vi "Action-engine-wrapper-example.vi"(7 "Action":T2(ring), 8 "error in (no error)":errorcluster, 9 "Additional message":string, 10 "Custom error":T1=enum."State not implemented") -> (0 "error out":errorcluster)   [LabVIEW 2013, in "Error-handling.lvlib" / "Errors.lvclass"]
uses:
  Errors.lvclass
  Custom-errors.ctl
  Settings.ctl
  Languages.ctl
  Ignore-error-custom.vi
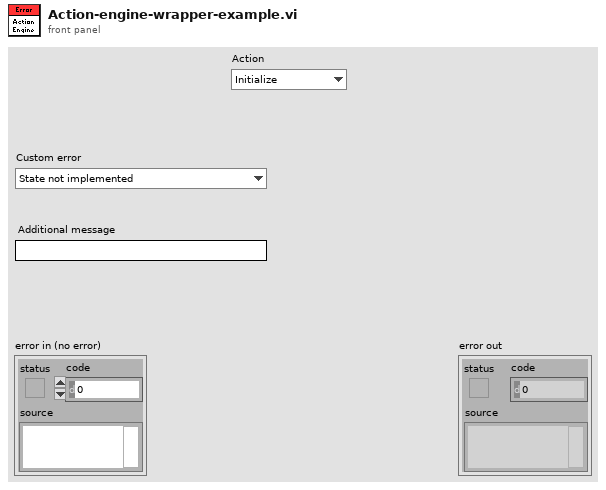
[diagram p1: front panel]
types:
  T1 = typedef "Error-handling.lvlib/Errors.lvclass/Custom-errors.ctl" = enum16{"No error", "State not implemented", "Initialization failed", "Language not implemented", "Error not implemented"}
  T2 = enum16{"Initialize", "Ignore", "Invoke", "Process", "Clear"}
  T3 = typedef "Error-handling.lvlib/Errors.lvclass/Settings.ctl" = cluster{"Language":T4, "Display error dialog":bool, "Write log to file":bool, "Stream to log file":bool, "Overwrite existing log":bool, "Max log size":i32, "Max number of log files":i32}
  T4 = typedef "Error-handling.lvlib/Errors.lvclass/Languages.ctl" = enum16{"English"}
  T5 = typedef "Error-handling.lvlib/Errors.lvclass/Object-reference.ctl" = refnum<data-value>
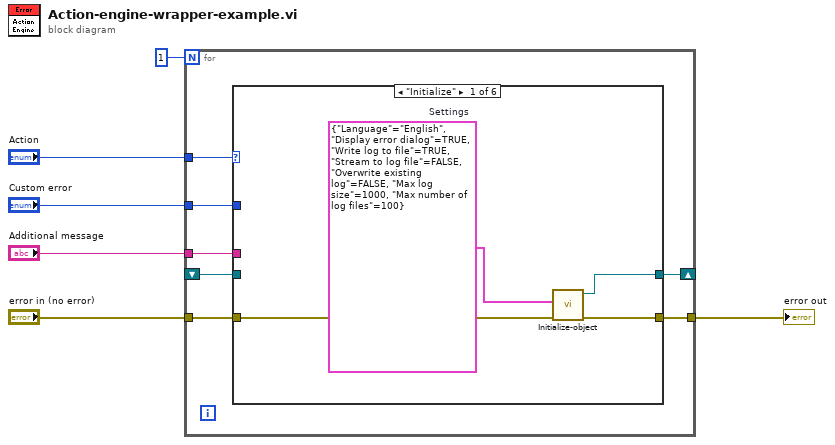
[diagram p0: block diagram]
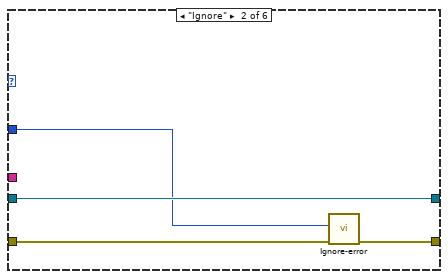
[diagram p2: hidden frame]
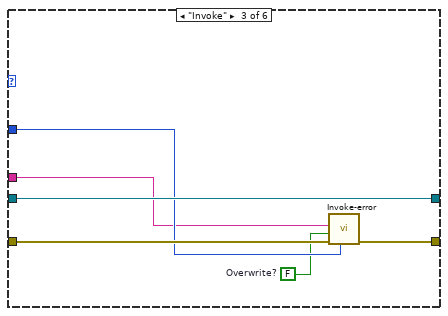
[diagram p3: hidden frame]
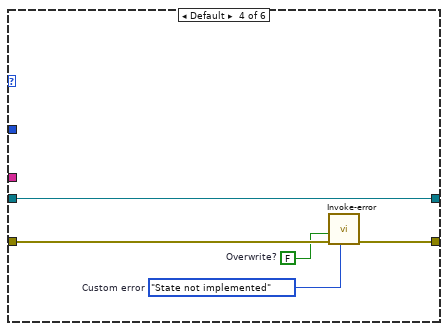
[diagram p4: hidden frame]
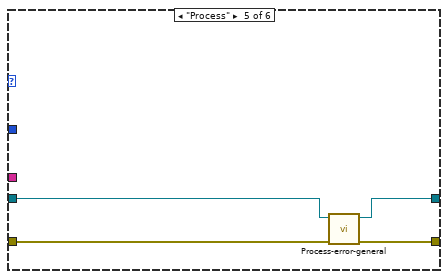
[diagram p5: hidden frame]
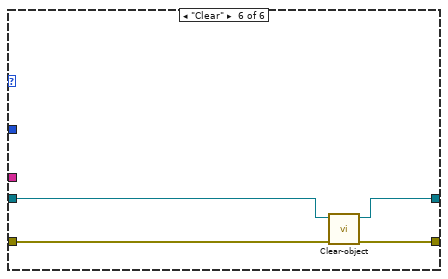
[diagram p6: hidden frame]
diagram:
  n1 = for {
    N: 1 -> [_]
    tunnel: "error in (no error)" -> [w10]
    tunnel: "Action" -> [w13]
    tunnel: "Custom error" -> [w12]
    tunnel: "Additional message" -> [w11]
    tunnel: [w9] -> w1
    shift-right: [w8] -> _
    shift-left: _ -> [w7]
    n2 = case shown="\"Initialize\"" w13 {
      tunnel: w12 -> [_ w18 w24 _ _ _]
      tunnel: w11 -> [_ _ w23 _ _ _]
      tunnel: w10 -> [w17 w19 w25 w30 w35 w39]
      tunnel: [w16 w21 w27 w32 w36 w40] -> w9
      tunnel: [w14 w20 w26 w31 w33 w37] -> w8
      tunnel: w7 -> [_ w20 w26 w31 w34 w38]
      frame "Initialize" {
        w15 = T3 {"Language"=enum."English", "Display error dialog"=TRUE, "Write log to file"=TRUE, "Stream to log file"=FALSE, "Overwrite existing log"=FALSE, "Max log size"=1000, "Max number of log files"=100}  # Settings
        n3 = call "Initialize-object.vi"("error in (no error)"=w17, "Settings"=w15) -> ("error out"=w16:errorcluster, "Errors out"=w14:T5)  [unwired: 8 in]
      }
      frame "Ignore" {
        n4 = call-poly "Ignore-error.vi"("error in (no error)"=w19, "Error to ignore"=w18) -> ("error out"=w21:errorcluster)  [unwired: 9 in]
      }
      frame "Invoke" {
        w22 = FALSE  # Overwrite?
        n5 = call "Invoke-error.vi"("Custom error"=w24, "error in (no error)"=w25, "Overwrite?"=w22, "Additional message"=w23) -> ("error out"=w27:errorcluster)  [unwired: 7 in]
      }
      frame Default {
        w28 = Custom-errors."State not implemented"  # Custom error
        w29 = FALSE  # Overwrite?
        n6 = call "Invoke-error.vi"("Custom error"=w28, "error in (no error)"=w30, "Overwrite?"=w29) -> ("error out"=w32:errorcluster)  [unwired: 8 in]
      }
      frame "Process" {
        n7 = call "Process-error-general.vi"("error in (no error)"=w35, "Errors in"=w34) -> ("error out"=w36:errorcluster, "Errors out"=w33:T5)  [unwired: 8 in]
      }
      frame "Clear" {
        n8 = call "Clear-object.vi"("error in (no error)"=w39, "Errors in"=w38) -> ("error out"=w40:errorcluster, "Errors out"=w37:T5)  [unwired: 8 in]
      }
    }
  }
  "error out" <- w1
